vi "pcfs_dither_loop_dither.vi"(8 "error in (no error)":errorcluster, 10 "first_dither?":bool, 11 "pcfs in":refnum<class "pcfs.lvclass">) -> (0 "error out":errorcluster, 3 "pcfs out":refnum<class "pcfs.lvclass">)   [LabVIEW 2015, in "pcfs.lvclass"]
uses:
  pcfs.lvclass
  pcfs.lvclass/pcfs.ctl
  Stage Class/Stage.lvclass
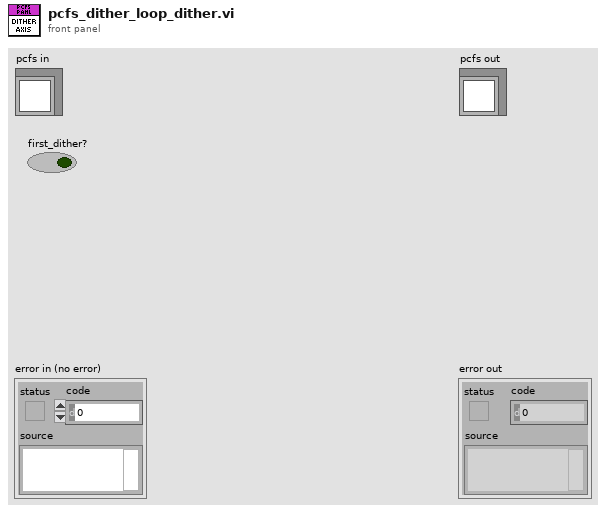
[diagram p1: front panel]
types:
  T1 = typedef "dither_trajectory_settings.ctl" = cluster{"PVT Ampl (nm)":dbl, "Dither Period (s)":dbl, "Type":T2, "Name":string}
  T2 = typedef "dither_trajectory_types.ctl" = enum16{"Sawtooth"}
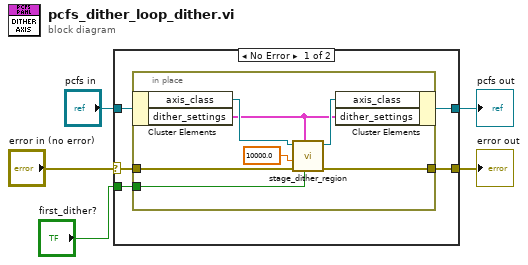
[diagram p0: block diagram]
diagram:
  n1 = case shown="No Error" "error in (no error)" {
    selector: "error in (no error)" -> [w9 w19]
    tunnel: [w8 w19] -> w4
    tunnel: [w7 w18] -> w2
    tunnel: "pcfs in" -> [w10 w18]
    tunnel: "first_dither?" -> [w6 _]
    frame No Error {
      n2 = in-place {
        in-place-border: w9 -> [w14]
        in-place-border: [w13] -> w8
        in-place-border: w6 -> [w11]
        n3 = in-place-cluster #1(w10) -> ("axis_class"=w16:refnum<class "Stage.lvclass">, "dither_settings"=w12:T1)
        n4 = call-dynamic "stage_dither_region.vi"("first_time?"=w11, "dither_params"=w12, "error in (no error)"=w14, "cycles"=10000.0, "Stage in"=w16) -> ("error out"=w13:errorcluster, "Stage out"=w15:refnum<class "Stage.lvclass">)  [unwired: 5 in]
        n5 = in-place-cluster #1("axis_class"=w15, "dither_settings"=w12) -> (w7:refnum<class "pcfs.lvclass">)
      }
    }
    frame Error {
    }
  }
  "error out" <- w4
  "pcfs out" <- w2
